vi "Example.vi"() -> ()   [LabVIEW 2018]
panel:
  out "Read Data":u8[](array[numeric])
  out "Read Count":i32
  out "Write Count":u16
  out "error IO":errorcluster
  in  "Data to Write":u8[](array[numeric])
  in  "Frequency Write":dbl
  in  "Reset":bool
  in  "VISA resource name":refnum<visa-resource-name>
  # "Autor: Gabriel Barbosa\nData: 08/06/2022\n\nObjetivo: \nDemonstar o uso do protocolo de comunicação\nLabView - Arduino. Antes de rodar a simulação, verifique as instruções\nde exemplo presentes na documentação referente ao Arduino. Note que \nesse protocolo não se restringe as placas Arduino, pode ser extendida para \nplacas de ESP32 e STM32, por exemplo. \nO objetivo dessa VI é demonstar o uso do protocolo. O usuário irá mandar \num vetor de 30 bytes do LabView e irá receber cada elemento desse vetor\nmultiplicado por dois."
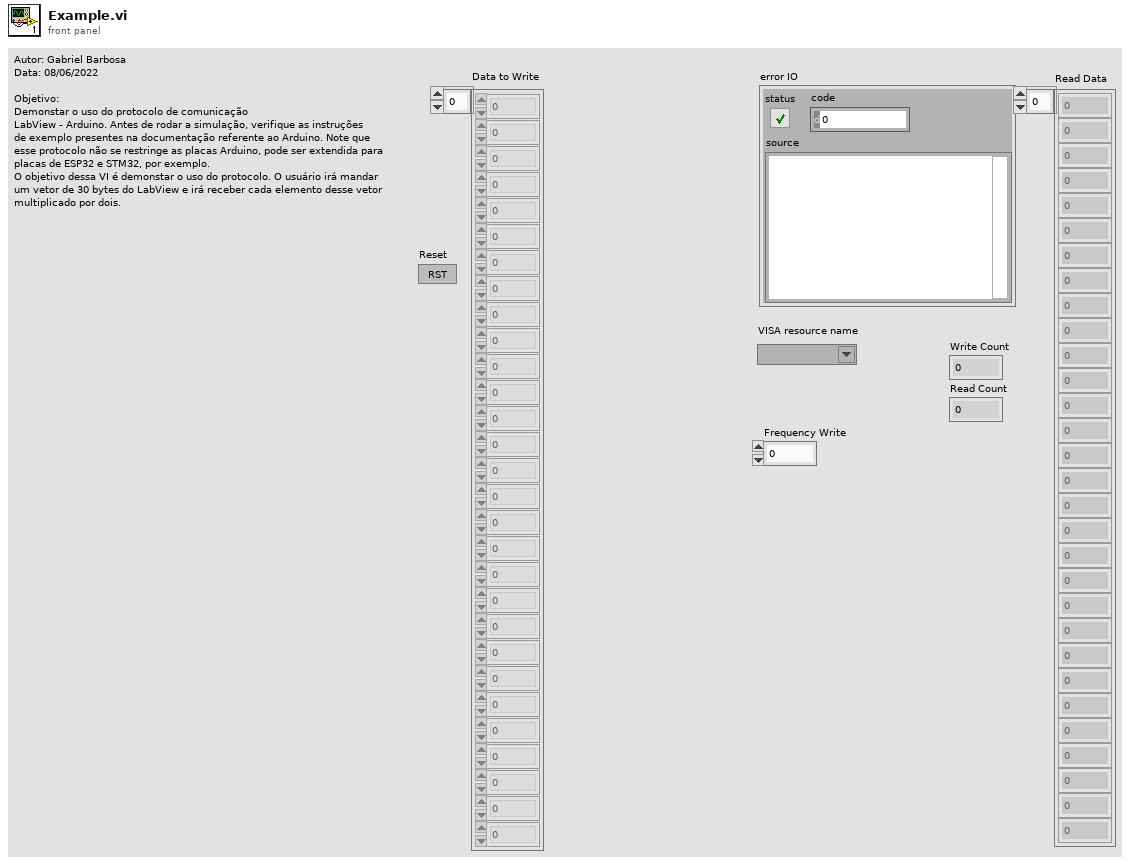
[diagram p1: front panel]
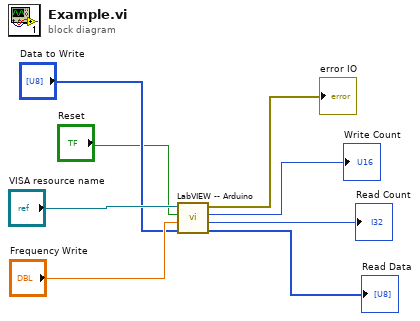
[diagram p0: block diagram]
diagram:
  n1 = call "LabVIEW -- Arduino.vi"("Data to Write"="Data to Write", "Frequency Write"="Frequency Write", "Reset"="Reset", "VISA resource name"="VISA resource name") -> ("Read Data"=→"Read Data":u8[], "Read Count"=→"Read Count":i32, "Write Count"=→"Write Count":u16, "error IO"=→"error IO":errorcluster)
